vi "FGV HoldingReg DBG.vi"() -> ()   [LabVIEW 2018, in "MB Relay.lvlib"]
uses:
  MB Relay.lvlib
  type defs/FGV enum.ctl
  type defs/MB relays _InstrumentType.ctl
panel:
  out "HoldingRegs":u16[](array[numeric])
  in  "stop":bool
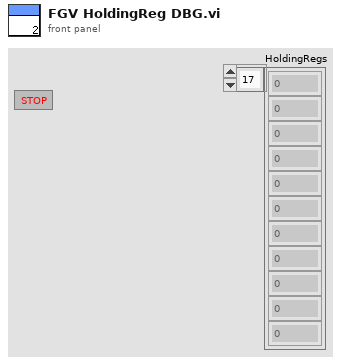
[diagram p1: front panel]
types:
  T1 = typedef "MB Relay.lvlib/MB relays _InstrumentType.ctl" = enum16{"JIG_TRIGGER", "JIG_RESET", "Relay SelfTest", "counter", "demux1_10(x6)", "mux10_1(x6)", "mux6_1(3wires)", "MB_Relay_01(eMICs)", "SpareRelays(DPDT)", "Optos", "Inputs", "DMM I 0.5", "SpareRelays (SPDT)", "SC enable"}
  T2 = typedef "MB Relay.lvlib/FGV enum.ctl" = enum16{"Write", "Init FGV", "Read", "All OFF", "All ON"}
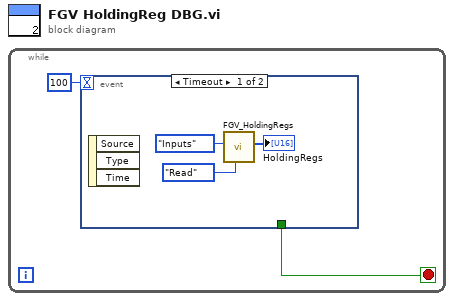
[diagram p0: block diagram]
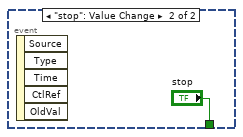
[diagram p2: hidden frame]
diagram:
  n1 = while {
    stop <- w1 stop-if-true
    n2 = event shown="[0] Timeout" {
      selector: _ -> [_ _]
      dyn-events: _ -> [_ _]
      timeout: 100 -> [_ _]
      tunnel: [_ "stop"] -> w1
      event Timeout {
        n3 = event-data() -> ()  [unwired: 1 in, 3 out]
        n4 = call "FGV_HoldingRegs.vi"("FGV_enum"=FGV_enum."Read", "Instruments"=MB_relays__InstrumentType."Inputs") -> ("HoldingRegs"=→"HoldingRegs":u16[])  [unwired: 7 in, 2 out]
      }
      event "stop": Value Change {
        n5 = event-data() -> ()  [unwired: 1 in, 5 out]
      }
    }
  }
